vi "Compensa Roda.vi"() -> ()   [LabVIEW 2016]
uses:
  <vilib>/Analysis/Matrix/Datatypes/RealMatrix.ctl
  <vilib>/Analysis/Matrix/Numeric/Multiply/Multiply - RM,RM.vi
  <vilib>/Analysis/Matrix/Numeric/Subtract/Subtract - RM,RM.vi
  <vilib>/Analysis/Matrix/Numeric/Conversions/Array To Matrix - RA.vi
  <vilib>/Analysis/baseanly.llb/Real Inverse Matrix.vi
  <vilib>/Analysis/Matrix/NI_Matrix.lvlib
  <vilib>/Analysis/NI_AALBase.lvlib
panel:
  in  "Roda Base":i32=3
  out "a":dbl
  in  "Velocidade do Robô Desejada":dbl[](array[numeric])=[0.0, 1.0, 0.0]
  in  "Velocidade das Rodas Lido":dbl[](array[numeric])=[0.866025, -0.866025, -0.707107, 0.1]
  out "Velocidade do Robô Obtida":T1
  out "Velocidade Necessária das Rodas":T1
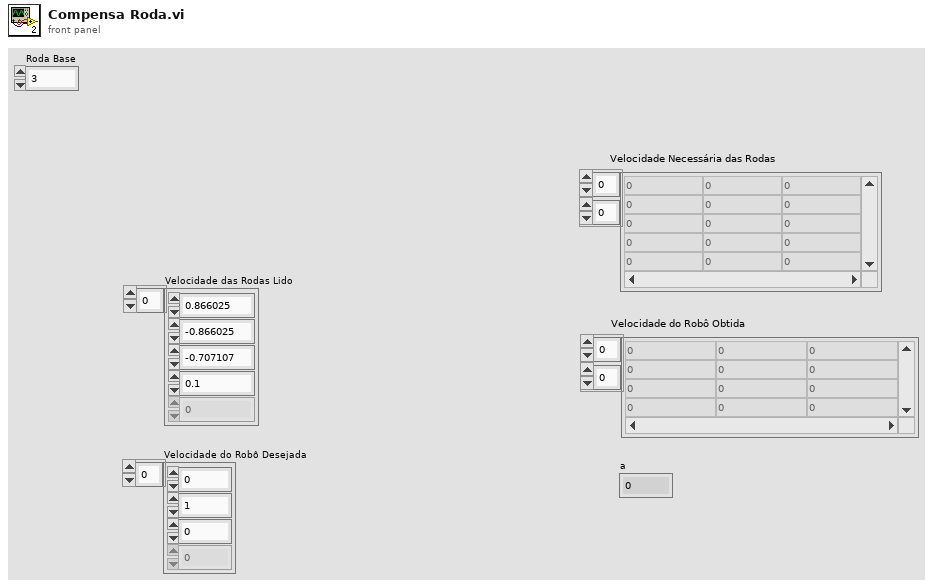
[diagram p1: front panel]
types:
  T1 = typedef "NI_Matrix.lvlib/RealMatrix.ctl" = dbl[][]
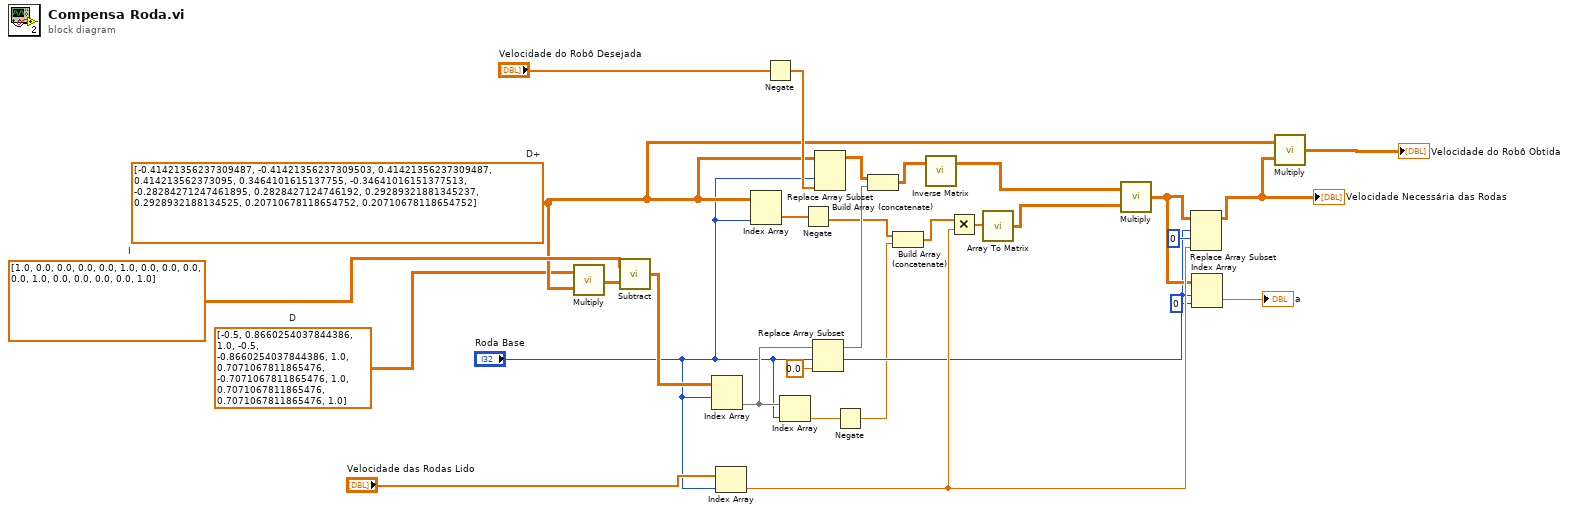
[diagram p0: block diagram]
diagram:
  w19 = T1 [[1.0, 0.0, 0.0, 0.0], [0.0, 1.0, 0.0, 0.0], [0.0, 0.0, 1.0, 0.0], [0.0, 0.0, 0.0, 1.0]]  # I
  w7 = T1 [[-0.5, 0.8660254037844386, 1.0], [-0.5, -0.8660254037844386, 1.0], [0.7071067811865476, -0.7071067811865476, 1.0], [0.7071067811865476, 0.7071067811865476, 1.0]]  # D
  w10 = T1 [[-0.41421356237309487, -0.41421356237309503, 0.41421356237309487, 0.414213562373095], [0.3464101615137755, -0.34641016151377513, -0.28284271247461895, 0.2828427124746192], [0.29289321881345237, 0.2928932188134525, 0.20710678118654752, 0.20710678118654752]]  # D+
  n1 = call-poly <vilib>:"Multiply.vi"("Real Matrix B"=w10, "Real Matrix A"=w7) -> ("A * B"=w20:T1)
  n2 = call-poly <vilib>:"Subtract.vi"("Real Matrix B"=w20, "Real Matrix A"=w19) -> ("A - B"=w18:T1)
  n3 = Index Array(array=w18, index (row)="Roda Base") -> (element=w26:dbl[])  [unwired: 1 in]
  n4 = Index Array(array="Velocidade das Rodas Lido", index="Roda Base") -> (element=w11:dbl)
  n5 = Index Array(array=w10, index (col)="Roda Base") -> (element=w24:dbl[])  [unwired: 1 in]
  n6 = Negate(x="Velocidade do Robô Desejada") -> (-x=w28:dbl[])
  n7 = Index Array(array=w26, index="Roda Base") -> (element=w2:dbl)
  n8 = Negate(x=w24) -> (-x=w14:dbl[])
  n9 = Replace Array Subset(array=w26, new element=0.0 ("new element/subarray"), index="Roda Base") -> (w16:dbl[])
  n10 = Replace Array Subset(array=w10, new element=w28, index (col)="Roda Base") -> (w17:T1)  [unwired: 1 in]
  n11 = Negate(x=w2) -> (-x=w1:dbl)
  n12 = Build Array (concatenate)(w17, w16) -> (w15:T1)
  n13 = Build Array (concatenate)(w14, w1) -> (w13:dbl[])
  n14 = call-poly <vilib>:"Inverse Matrix.vi"("Input Matrix"=w15) -> ("Inverse Matrix"=w27:T1)  [unwired: 1 in, 1 out]
  n15 = Multiply(x=w13, y=w11) -> (x*y=w22:dbl[])
  n16 = call-poly <vilib>:"Array To Matrix.vi"("Real 1D Array"=w22) -> ("Real Matrix (Column Vector)"=w21:T1)
  n17 = call-poly <vilib>:"Multiply.vi"("Real Matrix B"=w21, "Real Matrix A"=w27) -> ("A * B"=w6:T1)
  n18 = Replace Array Subset(array=w6, new element=w11, index (row)="Roda Base", index (col)=0 ("disabled index (col)")) -> (w9:T1)
  "Velocidade Necessária das Rodas" <- w9
  n19 = Index Array(array=w6, index (row)="Roda Base", index (col)=0 ("disabled index (col)")) -> (element=→"a":dbl)
  n20 = call-poly <vilib>:"Multiply.vi"("Real Matrix B"=w9, "Real Matrix A"=w10) -> ("A * B"=→"Velocidade do Robô Obtida":T1)
